vi "Check State-Value Table.vi"(8 "error in":errorcluster, 9 "state values":i32[](array[numeric]), 10 "state names":string[](array[string]), 11 "routing channel in":T1 format="%.0x") -> (0 "error out":errorcluster, 3 "routing channel out":T1=18446744073709551615 format="%.0x")   [LabVIEW 2020, in "Routing and Faulting Scripting.lvlib"]
uses:
  Routing and Faulting Scripting.lvlib
  <vilib>/NI VeriStand/Custom Device API/Custom Device Item Ref.ctl
  <vilib>/NI VeriStand/Custom Device API/Custom Device API.lvlib
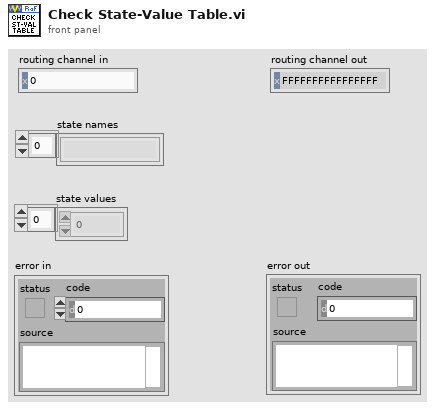
[diagram p1: front panel]
types:
  T1 = typedef "Custom Device API.lvlib/Custom Device Item Ref.ctl" = u64
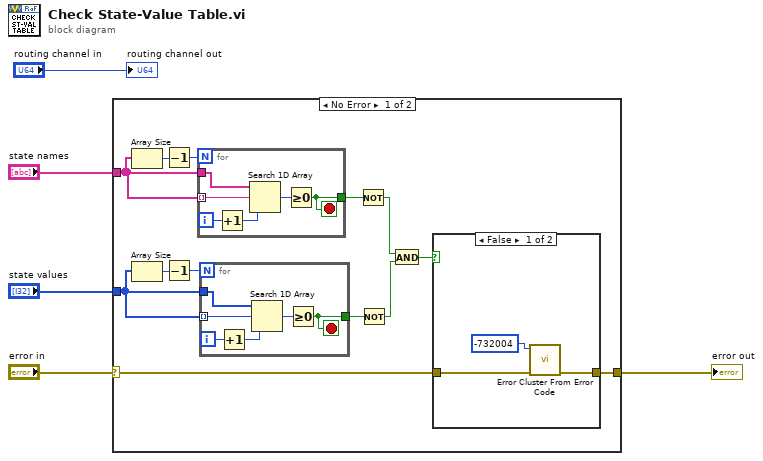
[diagram p0: block diagram]
diagram:
  n1 = case shown="No Error" "error in" {
    selector: "error in" -> [w18 w35]
    tunnel: [w17 w35] -> w4
    tunnel: "state names" -> [w12 _]
    tunnel: "state values" -> [w6 _]
    frame No Error {
      n2 = Array Size(array=w12) -> (size(s)=w10:i32)
      n3 = Array Size(array=w6) -> (size(s)=w8:i32)
      n4 = Decrement(x=w10) -> (x-1=w11:i32)
      n5 = Decrement(x=w8) -> (x-1=w7:i32)
      n6 = for {
        N: w11 -> [_]
        tunnel: [w33] -> w15
        tunnel: w12 -> [w31] mode=indexing
        tunnel: w12 -> [w30]
        i -> [w32]
        stop <- w33 stop-if-true
        n7 = Increment(x=w32) -> (x+1=w29:i32)
        n8 = Search 1D Array(1D array=w30, element=w31, start index (0)=w29) -> (index of element=w34:i32)
        n9 = Greater Or Equal To 0?(x=w34) -> (x >= 0?=w33:bool)
      }
      n10 = for {
        N: w7 -> [_]
        tunnel: [w23] -> w9
        tunnel: w6 -> [w21] mode=indexing
        tunnel: w6 -> [w20]
        i -> [w22]
        stop <- w23 stop-if-true
        n11 = Increment(x=w22) -> (x+1=w19:i32)
        n12 = Search 1D Array(1D array=w20, element=w21, start index (0)=w19) -> (index of element=w24:i32)
        n13 = Greater Or Equal To 0?(x=w24) -> (x >= 0?=w23:bool)
      }
      n14 = Not(x=w15) -> (.not. x?=w14:bool)
      n15 = Not(x=w9) -> (.not. x?=w13:bool)
      n16 = And(x=w14, y=w13) -> (x .and. y?=w16:bool)
      n17 = case shown="False" w16 {
        tunnel: w18 -> [w25 w28]
        tunnel: [w26 w28] -> w17
        frame False {
          n18 = call <vilib>:"Error Cluster From Error Code.vi"("error in (no error)"=w25, "error code (0)"=-732004) -> ("error out"=w26:errorcluster)  [unwired: 7 in]
        }
        frame True {
        }
      }
    }
    frame Error {
    }
  }
  "error out" <- w4
  "routing channel out" <- "routing channel in"
